vi "refresh.vi"(8 "error in (no error)":errorcluster, 10 "Engine Configuration In":refnum<class "engine configuration.lvclass">, 11 "E2E Tag Exchange editor node In":refnum<class "E2E Tag Exchange editor node.lvclass">) -> (0 "error out":errorcluster, 2 "Engine Configuration Out":refnum<class "engine configuration.lvclass">, 3 "E2E Tag Exchange editor node Out":refnum<class "E2E Tag Exchange editor node.lvclass">)   [LabVIEW 2015, in "E2E Tag Exchange editor node.lvclass"]
uses:
  E2E Tag Exchange editor node.lvclass
  <vilib>/NI/Module Execution Interface/Engine Configuration/engine configuration.lvclass
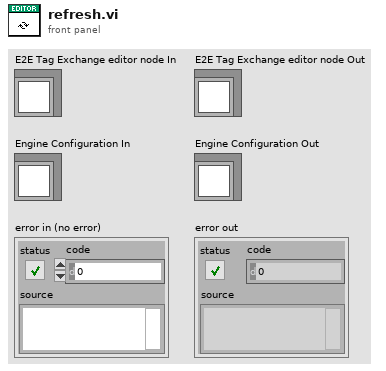
[diagram p1: front panel]
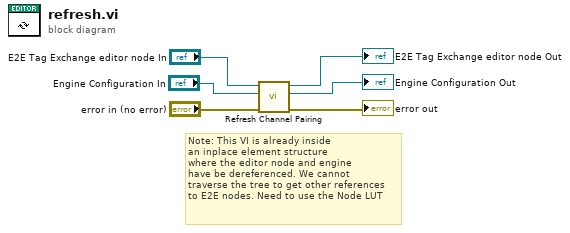
[diagram p0: block diagram]
diagram:
  # "Note: This VI is already inside\nan inplace element structure\nwhere the editor node and engine\nhave be dereferenced. We cannot\ntraverse the tree to get other references\nto E2E nodes. Need to use the Node LUT"
  n1 = call "Refresh Channel Pairing.vi"("error in (no error)"="error in (no error)", "engine configuration in"="Engine Configuration In", "E2E editor node in"="E2E Tag Exchange editor node In") -> ("error out"=→"error out":errorcluster, "engine configuration out"=→"Engine Configuration Out":refnum<class "engine configuration.lvclass">, "E2E editor node out"=→"E2E Tag Exchange editor node Out":refnum<class "E2E Tag Exchange editor node.lvclass">)  [unwired: 6 in]
